vi "GFITS_SetImname.vi"(8 "error in (no error)":errorcluster, 10 "name":string, 11 "Database RefNum":T1) -> (0 "error out":errorcluster)   [LabVIEW 2016]
uses:
  DBSHAND/private/vis/DatabaseHand_RefNum.ctl
  DBSHAND/private/vis/DatabaseHand_Element_Set(string).vi
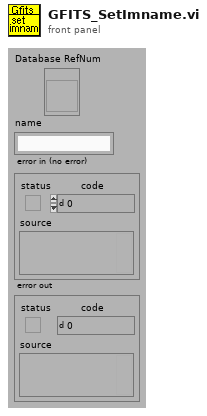
[diagram p1: front panel]
types:
  T1 = typedef "DatabaseHand_RefNum.ctl" = refnum<vi>
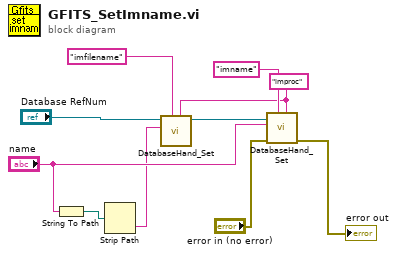
[diagram p0: block diagram]
diagram:
  w5 = "improc" ("group")
  n1 = String To Path(string="name") -> (path=w2:path)
  n2 = Strip Path(path=w2) -> (name=w1:string)  [unwired: 1 out]
  n3 = call-poly "DatabaseHand_Set.vi"("group"=w5, "name"="imfilename", "value"=w1, "Database RefNum in"="Database RefNum") -> ("Database RefNum out"=w6:T1)  [unwired: 4 in, 3 out]
  n4 = call-poly "DatabaseHand_Set.vi"("group"=w5, "name"="imname", "error in (no error)"="error in (no error)", "value"="name", "Database RefNum in"=w6) -> ("error out"=→"error out":errorcluster)  [unwired: 3 in, 3 out]
